vi "gwyscan add gwyddion array.vi"(0 "data":dbl[](array[numeric]), 1 "xres":i32, 2 "yres":i32, 3 "xreal":dbl, 4 "yreal":dbl, 5 "xyunit":string, 6 "zunit":string, 7 "error in (no error)":errorcluster, 8 "description":string, 9 "filename":string) -> (18 "description out":string, 19 "filename out":string, 20 "data OUT":dbl[](array[numeric]), 21 "function return":i32, 25 "xyunit out":string, 26 "zunit out":string, 27 "error out":errorcluster)   [LabVIEW 2016, in "libgwyscan.lvlib"]
doc: "GWYSCANDLL_API int gwyscan_add_gwyddion_array(double *data, int xres, int yres, double xreal, double yreal, char *xyunit, char *zunit, char *description, char *filename);\n\nGWYSCANDLL_API GwyscanResult gwyscan_add_gwyddion_array(const double *data, int xres, int yres, double xreal, double yreal, const char *xyunit, const char *zunit, const char *description, const char *filename);"
uses:
  libgwyscan.lvlib
  libgwyscan.dll
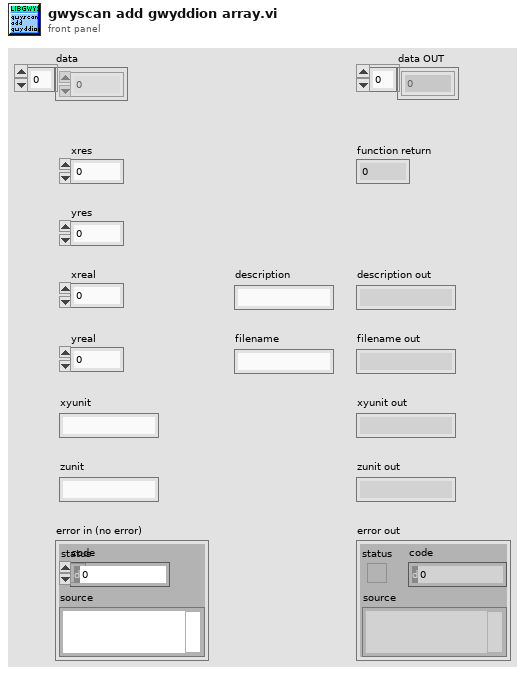
[diagram p1: front panel]
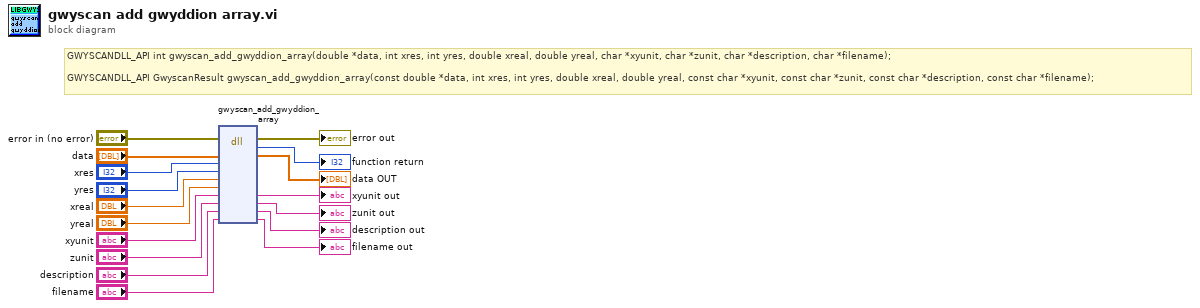
[diagram p0: block diagram]
diagram:
  # "GWYSCANDLL_API int gwyscan_add_gwyddion_array(double *data, int xres, int yres, double xreal, double yreal, char *xyunit, char *zunit, char *description, char *filename);\n\nGWYSCANDLL_API GwyscanResult gwyscan_add_gwyddion_array(const double *data, int xres, int yres, double xreal, double yreal, const char *xyunit, const char *zunit, const char *description, const char *filename);"
  n1 = dll-call lib="PTH2’abs CUsersCharlÃ¨ne BrillardDesktoplbni-lbniAFMController-BetaVersionv2.0.16-20190611 libgwyscan-1.2-labview2015-win32libgwyscan.dll" fn="gwyscan_add_gwyddion_array"(error in="error in (no error)", "data"="data", "xres"="xres", "yres"="yres", "xreal"="xreal", "yreal"="yreal", "xyunit"="xyunit", "zunit"="zunit", "description"="description", "filename"="filename") -> (error out=→"error out":errorcluster, "return type"=→"function return":i32, "data"=→"data OUT":dbl[], "xyunit"=→"xyunit out":string, "zunit"=→"zunit out":string, "description"=→"description out":string, "filename"=→"filename out":string)  [unwired: 6 in, 1 out]
